vi "Write FlexLogger Data.vi"() -> ()   [LabVIEW 2024]
doc: "Demonstrates how to use network streams to pass data and commands between two running VIs. It displays waveform data that is received from the target VI and sends commands to update the frequency of the generated signal."
uses:
  <resource>/objmgr/ni.dex.rc
panel:
  in  "stop":bool
  out "Data":waveform(dbl)[](graph)
  # "Overview: Demonstrates how to use Network Streams to write data to the FlexLogger StreamReader plug-in.\nRequirements: Windows\nInstructions:\n1. Run this VI.\n2. Build and insert the StreamReader plug-in in FlexLogger.\n3. Click Stop to stop the VI."
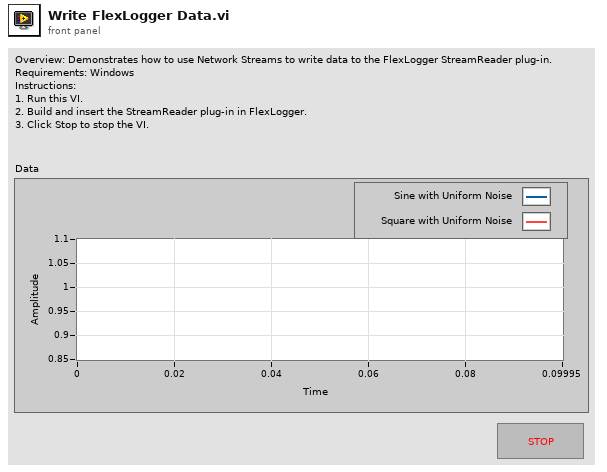
[diagram p1: front panel]
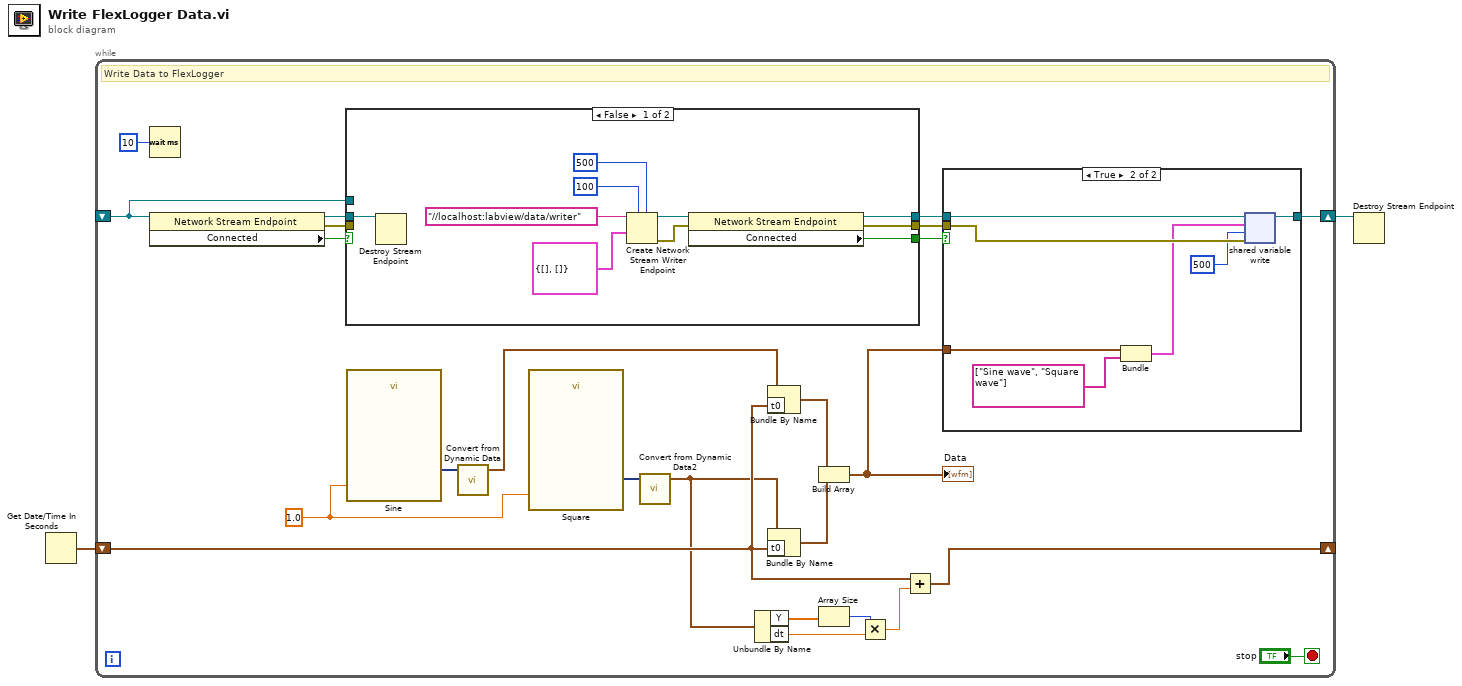
[diagram p0: block diagram]
diagram:
  n1 = Get Date/Time In Seconds() -> (seconds since 1Jan1904=w1:timestamp)
  n2 = while "Target->Host Data Reader" {
    shift-right: [w20] -> w2
    shift-left: _ -> [w16]
    shift-right: [w3] -> _
    shift-left: w1 -> [w9]
    stop <- "stop" stop-if-true
    w24 = 1.0
    # "Write Data to FlexLogger"
    n3 = Wait (ms)(milliseconds to wait=u32 10) -> ()  [unwired: 1 out]
    n4 = property class="Network Stream Endpoint"(reference=w16) -> (reference out=w17:refnum<k21>, error out=w19:errorcluster, "Connected"=w18:bool)  [unwired: 1 in]
    n5 = case shown="False" w18 {
      selector: w18 -> [_ w37]
      tunnel: [w36 w38] -> w14
      tunnel: [w31 w39] -> w15
      tunnel: w17 -> [w35 w39]
      tunnel: [w34 w37] -> w13
      tunnel: w19 -> [_ w38]
      tunnel: w16 -> [_ _]
      frame False {
        n6 = Destroy Stream Endpoint(11:w35) -> ()  [unwired: 1 in, 1 out]
        n7 = Create Network Stream Writer Endpoint(5:500 ("timeout in ms (-1)"), 7:100 ("writer buffer size"), 9:cluster{waveform(dbl)[], string[]} {[], []} ("output cluster"), 11:"//localhost:labview/data/writer" ("writer name")) -> (0:w32:errorcluster, 3:w33:refnum<k21>)  [unwired: 3 in]
        n8 = property class="Network Stream Endpoint"(reference=w33, error in=w32) -> (reference out=w31:refnum<k21>, error out=w36:errorcluster, "Connected"=w34:bool)
      }
      frame True {
      }
    }
    n9 = call "Sine"("Frequency"=w24) -> ("Sine with Uniform Noise"=w25:dynamicdata)  [unwired: 13 in, 1 out]
    n10 = call "Convert from Dynamic Data"("Dynamic Data Type"=w25) -> ("Waveform"=w11:waveform(dbl))  [unwired: 3 in]
    n11 = call "Square"("Frequency"=w24) -> ("Square with Uniform Noise"=w26:dynamicdata)  [unwired: 13 in, 1 out]
    n12 = call "Convert from Dynamic Data2"("Dynamic Data Type"=w26) -> ("Waveform"=w8:waveform(dbl))  [unwired: 3 in]
    n13 = Unbundle By Name(w8) -> ("Y"=w7:dbl[], "dt"=w5:dbl)
    n14 = Bundle By Name(cluster=w11, "t0"=w9) -> (w12:waveform(dbl))
    n15 = Bundle By Name(cluster=w8, "t0"=w9) -> (w10:waveform(dbl))
    n16 = Build Array(w12, w10) -> (w23:waveform(dbl)[])
    "Data" <- w23
    n17 = Array Size(array=w7) -> (size(s)=w6:i32)
    n18 = Multiply(x=w6, y=w5) -> (x*y=w4:dbl)
    n19 = Add(x=w9, y=w4) -> (x+y=w3:timestamp)
    n20 = case shown="True" w13 {
      tunnel: w15 -> [w40 w47]
      tunnel: w14 -> [_ w46]
      tunnel: [w40 w45] -> w20
      tunnel: w23 -> [_ w43]
      frame False {
      }
      frame True {
        n21 = Bundle(w43, string[] ["Sine wave", "Square wave"]) -> (w42:cluster{waveform(dbl)[], string[]})  [unwired: 1 in]
        n22 = shared-variable-write(w47, w46, w42, 500 ("timeout ms (-1)")) -> (w45:refnum<k21>)  [unwired: 2 out]
      }
    }
  }
  n23 = Destroy Stream Endpoint(11:w2) -> ()  [unwired: 1 in, 1 out]
